vi "USRP_TXInit.vi"(0 "device names":refnum<k15>, 1 "USRP ControledParameters":T1={"active antenna"="TX1", "gain"=0.0, "carrier frequency"=100000.0, "IQ rate"=100000.0} {"IQ rate" format="%#_6p"; "carrier frequency" format="%#_6p"; "gain" format="%#_6f"}, 3 "error in (no error)":errorcluster) -> (7 "session handle out":refnum<k15>, 8 "USRP CoercedParamters":T2={"coerced IQ rate"=100000.0, "coerced carrier frequency"=100000.0, "coerced gain"=0.0} {"coerced gain" format="%#_6f"; "coerced carrier frequency" format="%#_6p"; "coerced IQ rate" format="%#_6p"}, 10 "error out":errorcluster)   [LabVIEW 2022 SP3]
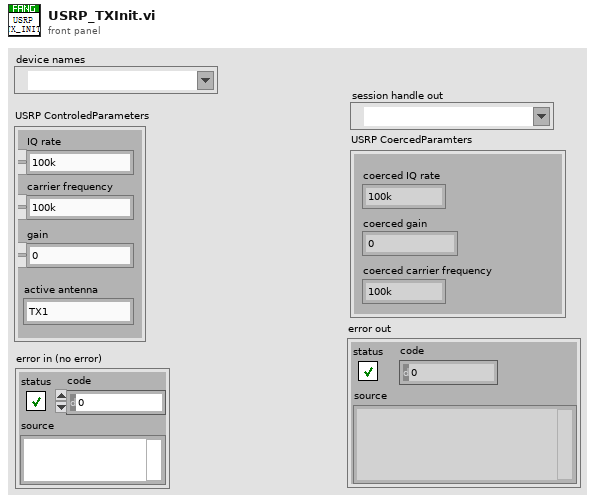
[diagram p1: front panel]
types:
  T1 = cluster{"active antenna":string, "gain":dbl, "carrier frequency":dbl, "IQ rate":dbl}
  T2 = cluster{"coerced IQ rate":dbl, "coerced carrier frequency":dbl, "coerced gain":dbl}
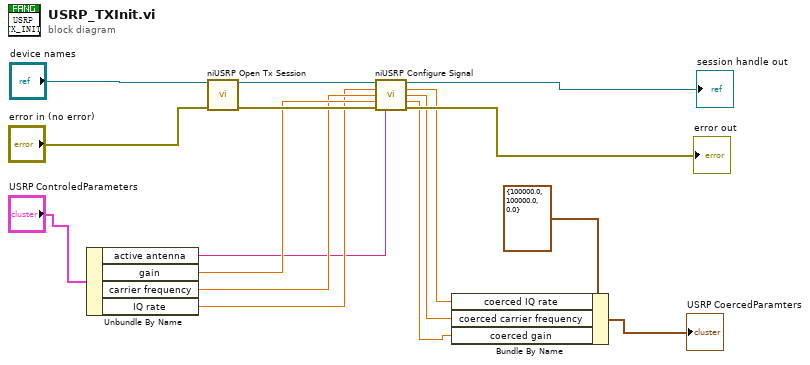
[diagram p0: block diagram]
diagram:
  n1 = Unbundle By Name("USRP ControledParameters") -> ("active antenna"=w1:string, "gain"=w10:dbl, "carrier frequency"=w9:dbl, "IQ rate"=w8:dbl)
  n2 = call <instrlib>:"niUSRP Open Tx Session.vi"("device names"="device names", "error in (no error)"="error in (no error)") -> ("session handle out"=w16:refnum<k15>, "error out"=w11:errorcluster)  [unwired: 12 in]
  n3 = call <instrlib>:"niUSRP Configure Signal.vi"("session handle"=w16, "IQ rate"=w8, "carrier frequency"=w9, "gain"=w10, "error in (no error)"=w11, "active antenna"=w1) -> ("session handle out"=→"session handle out":refnum<k15>, "coerced IQ rate"=w6:dbl, "coerced carrier frequency"=w5:dbl, "coerced gain"=w4:dbl, "error out"=→"error out":errorcluster)  [unwired: 5 in]
  n4 = Bundle By Name(cluster=T2 {"coerced IQ rate"=100000.0, "coerced carrier frequency"=100000.0, "coerced gain"=0.0} ("USRP CoercedParamters"), "coerced IQ rate"=w6, "coerced carrier frequency"=w5, "coerced gain"=w4) -> (→"USRP CoercedParamters":T2)
